vi "Stop.vi"(8 "error in (no error)":errorcluster, 10 "Message in":refnum<class "StopMessage.lvclass">, 11 "Galvo in":refnum<class "ImagingModeSPIM.lvclass">) -> (0 "error out":errorcluster, 3 "Galvo out":refnum<class "ImagingModeSPIM.lvclass">)   [LabVIEW 2012, in "ImagingModeSPIM.lvclass"]
doc: "This member function is called when the statemachine in the run.vi receives an 'stop' command. It relays the message to all observers of the component.\n\nOverride this member function in your derived class if you need additional stop functionality (but don't forget to call the parent method)."
uses:
  ImagingModeSPIM.lvclass
  <vilib>/Distrio/Murmex/StopMessage/StopMessage.lvclass
  <vilib>/Distrio/Murmex/Murmex/Murmex.lvclass
  ImagingModeSPIM.lvclass/ImagingModeSPIM.ctl
panel:
  # "This method is called when the STOP\ntrigger is sent. \n\nOverride this method when your component needs to\nrespond to this trigger. \n\nCall parent for proper implementation"
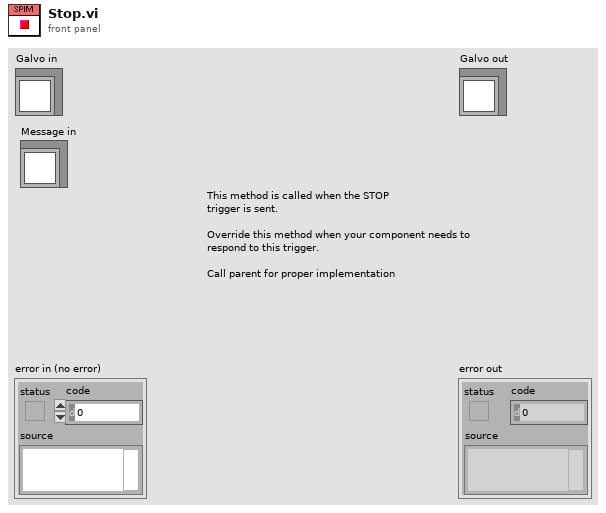
[diagram p1: front panel]
types:
  T1 = enum8{"Enabled", "Disabled", "Disabled and Grayed Out"}
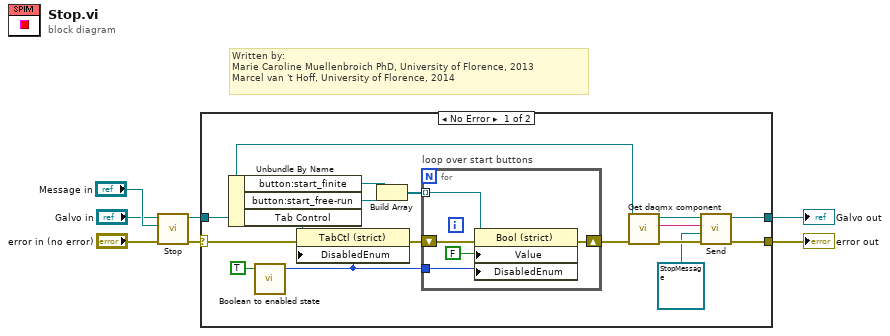
[diagram p0: block diagram]
diagram:
  # "Written by:\nMarie Caroline Muellenbroich PhD, University of Florence, 2013 \nMarcel van 't Hoff, University of Florence, 2014"
  n1 = call-parent "Stop.vi"("error in (no error)"="error in (no error)", "Message in"="Message in", "Murmex in"="Galvo in") -> ("error out"=w4:errorcluster, "Murmex out"=w3:refnum<class "ImagingModeSPIM.lvclass">)  [unwired: 7 in]
  n2 = case shown="No Error" w4 {
    selector: w4 -> [w17 w29]
    tunnel: w3 -> [w12 w30]
    tunnel: [w10 w30] -> w2
    tunnel: [w14 w29] -> w1
    frame No Error {
      n3 = Unbundle By Name(w12) -> ("button:start_finite"=w23:refnum<vi>, "button:start_free-run"=w22:refnum<vi>, "Tab Control"=w18:refnum<vi>)
      n4 = call <vilib>:"Boolean to enabled state.vi"("boolean in"=TRUE) -> ("enabled status out"=w15:T1)  [unwired: 4 in]
      n5 = property class="TabCtl (strict)"(reference=w18, error in=w17, "DisabledEnum"=w15) -> (error out=w16:errorcluster)  [unwired: 1 out]
      n6 = Build Array(w23, w22) -> (w21:refnum<vi>[])
      n7 = for "loop over start buttons" {
        tunnel: w21 -> [w28] mode=indexing
        shift-right: [w26] -> w20
        shift-left: w16 -> [w27]
        tunnel: w15 -> [w24]
        n8 = property class="Bool (strict)"(reference=w28, error in=w27, "Value"=FALSE, "DisabledEnum"=w24) -> (error out=w26:errorcluster)  [unwired: 1 out]
      }
      n9 = call-dynamic "Get daqmx component.vi"("error in (no error)"=w20, "ImagingModeSPIM in"=w12) -> ("error out"=w13:errorcluster, "daqmx component"=w9:string, "ImagingModeSPIM out"=w11:refnum<class "ImagingModeSPIM.lvclass">)  [unwired: 7 in]
      n10 = call <vilib>:"Send.vi"("error in (no error)"=w13, "Message"=refnum<class "StopMessage.lvclass"> refnum ("Distrio Murmex 1.5:StopMessage"), "recipient"=w9, "Murmex in"=w11) -> ("error out"=w14:errorcluster, "Murmex out"=w10:refnum<class "ImagingModeSPIM.lvclass">)  [unwired: 6 in]
    }
    frame Error {
    }
  }
  "error out" <- w1
  "Galvo out" <- w2
